vi "Resize Rendezvous.vi"(8 "error in (no error)":errorcluster, 9 "Threads":i32, 10 "Rendezvous Index":i32, 11 "System Actor in":refnum<class "System Actor.lvclass">) -> (0 "error out":errorcluster, 3 "System Actor out":refnum<class "System Actor.lvclass">)   [LabVIEW 2024, in "System Actor.lvclass"]
uses:
  System Actor.lvclass
  System Actor.lvclass/System Actor.ctl
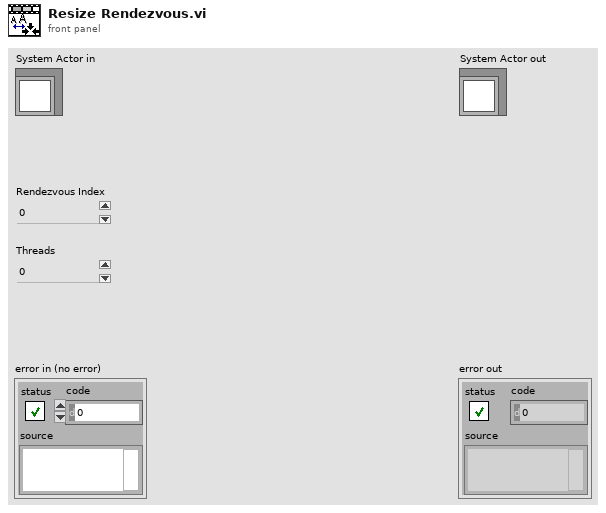
[diagram p1: front panel]
types:
  T1 = typedef "Rendezvous RefNum" = refnum<k1>
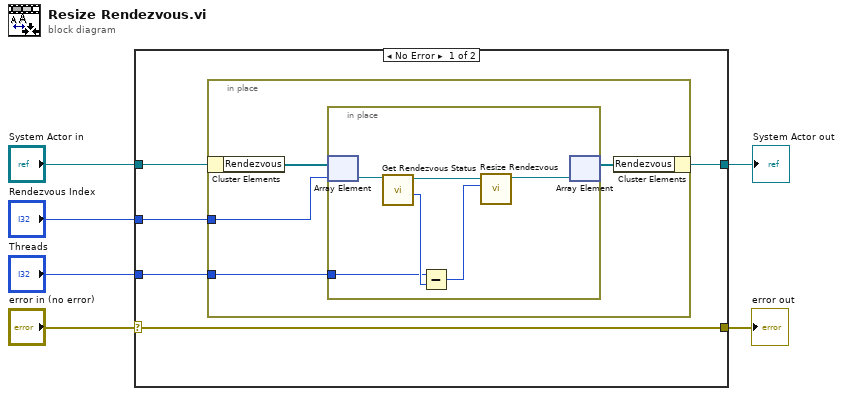
[diagram p0: block diagram]
diagram:
  n1 = case shown="No Error" "error in (no error)" {
    selector: "error in (no error)" -> [w11 w23]
    tunnel: [w11 w23] -> w5
    tunnel: [w9 w22] -> w3
    tunnel: "System Actor in" -> [w10 w22]
    tunnel: "Rendezvous Index" -> [w8 _]
    tunnel: "Threads" -> [w7 _]
    frame No Error {
      n2 = in-place {
        in-place-border: w8 -> [w14]
        in-place-border: w7 -> [w12]
        n3 = in-place-cluster #1(w10) -> ("Rendezvous"=w15:T1[])
        n4 = in-place {
          in-place-border: w12 -> [w19]
          n5 = in-place-array #2(w15, w14) -> (w21:T1)
          n6 = call <vilib>:"Get Rendezvous Status.vi"("rendezvous"=w21) -> ("size"=w20:i32, "rendezvous out"=w16:T1)  [unwired: 6 in, 3 out]
          n7 = Subtract(x=w19, y=w20) -> (x-y=w17:i32)
          n8 = call <vilib>:"Resize Rendezvous.vi"("size change (0)"=w17, "rendezvous"=w16) -> ("rendezvous out"=w18:T1)  [unwired: 3 in, 2 out]
          n9 = in-place-array #2(w18) -> (w13:T1[])  [unwired: 1 out]
        }
        n10 = in-place-cluster #1("Rendezvous"=w13) -> (w9:refnum<class "System Actor.lvclass">)
      }
    }
    frame Error {
    }
  }
  "error out" <- w5
  "System Actor out" <- w3
